vi "IR Emitter Test.vi"(5 "Test Config":T1={"Chopper RPM"=140, "IR Power"=5, "Conc Tolerance"=0.0, "Gas Stable Time"=0, "A-D Settle"=0, "Samples"=0, "Filter Time"=0, "Gas Mixtures"=[], "Filter Sequences"=[], "Functional Test"={"Mic Test ON ADC Max"=0.0, "Mic Test ON ADC Min"=0.0, "Mic Test OFF ADC Max"=0.0, "Mic Test OFF ADC Min"=0.0, "Mic Test IC ADC Max"=0.0, "Mic Test IC ADC Min"=0.0, "IR Emitter ON ADC Max"=0.0, "IR Emitter ON ADC Min"=0.0, "IR Emitter OFF ADC Max"=0.0, "IR Emitter OFF ADC Min"=0.0}, "Initial Flow Rate"=0.0, "Max Flow Rate"=0.0} {"Gas Mixtures"."ADC Gains" items=["0"=0, "3"=3, "4"=4, "5"=5, "6"=6, "7"=7]; "Conc Tolerance" min=0.0 max=100.0 step=1.0; "IR Power" min=2 max=5 step=1; "Chopper RPM" min=140 max=1000 step=1}, 8 "error in (no error)":errorcluster, 11 "Session Handle in":T6) -> (0 "error out":errorcluster, 1 "Failure Reason":string, 2 "Passed?":bool, 3 "Session Handle out":T6)   [LabVIEW 2015, in "PAS.lvclass"]
uses:
  PAS.lvclass
  Typedefs/Session Handle.ctl
  Tests/Controls/Test Config.ctl
  Tests/Controls/Gas Mixture.ctl
  Typedefs/ADC Gains.ctl
  Tests/Controls/Filter Sequence.ctl
  Tests/Controls/Functional Test.ctl
  Typedefs/Emitter Power.ctl
  Typedefs/Valves.ctl
panel:
  out "Passed?":bool
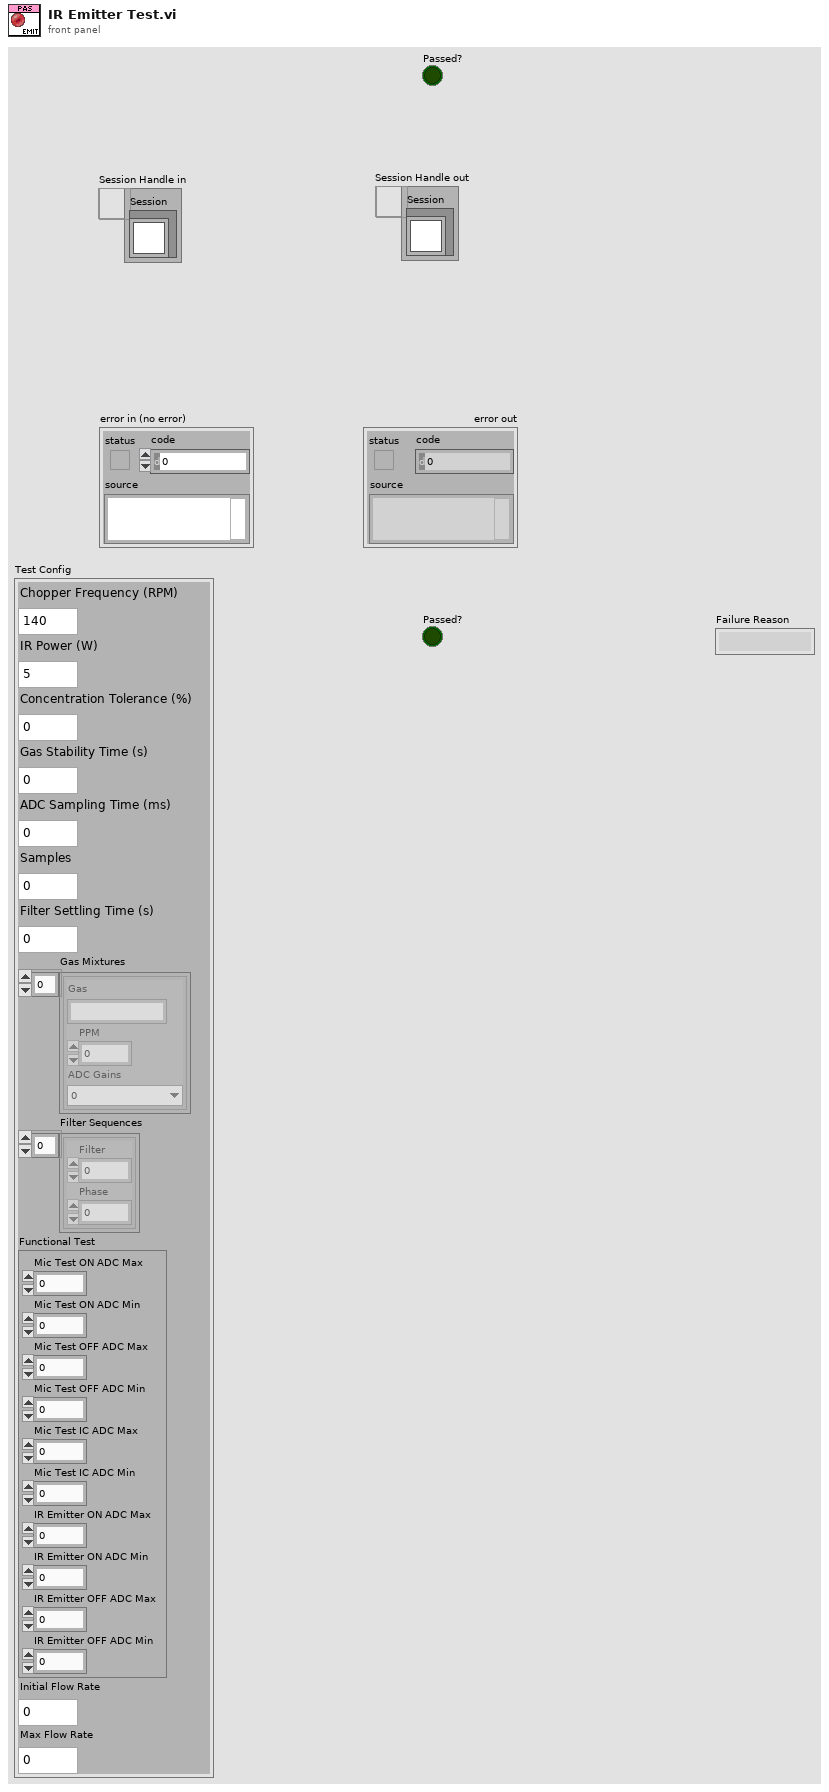
[diagram p1: front panel]
types:
  T1 = typedef "Test Config.ctl" = cluster{"Chopper RPM":u16, "IR Power":u8, "Conc Tolerance":dbl, "Gas Stable Time":u16, "A-D Settle":u16, "Samples":u16, "Filter Time":u16, "Gas Mixtures":T2[], "Filter Sequences":T4[], "Functional Test":T5, "Initial Flow Rate":sgl, "Max Flow Rate":sgl}
  T2 = typedef "Gas Mixture.ctl" = cluster{"Gas":string, "PPM":dbl, "ADC Gains":T3}
  T3 = typedef "PAS.lvclass/ADC Gains.ctl" = u16
  T4 = typedef "Filter Sequence.ctl" = cluster{"Filter":u8, "Phase":dbl}
  T5 = typedef "Functional Test.ctl" = cluster{"Mic Test ON ADC Max":dbl, "Mic Test ON ADC Min":dbl, "Mic Test OFF ADC Max":dbl, "Mic Test OFF ADC Min":dbl, "Mic Test IC ADC Max":dbl, "Mic Test IC ADC Min":dbl, "IR Emitter ON ADC Max":dbl, "IR Emitter ON ADC Min":dbl, "IR Emitter OFF ADC Max":dbl, "IR Emitter OFF ADC Min":dbl}
  T6 = typedef "PAS.lvclass/Session Handle.ctl" = refnum<data-value>
  T7 = typedef "PAS.lvclass/Valves.ctl" = u16
  T8 = typedef "PAS.lvclass/Emitter Power.ctl" = u16
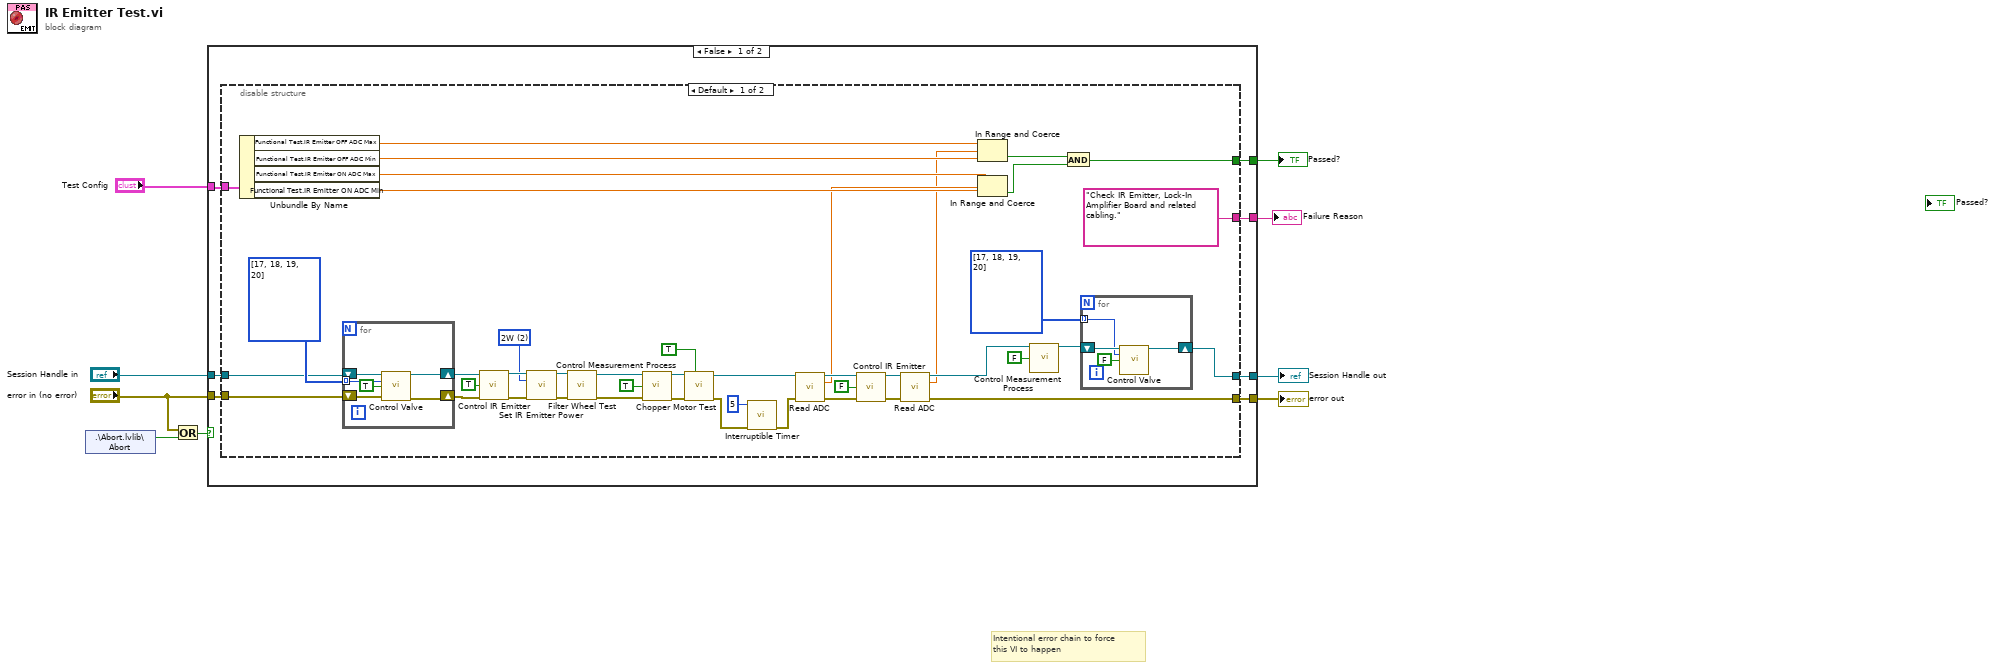
[diagram p0: block diagram]
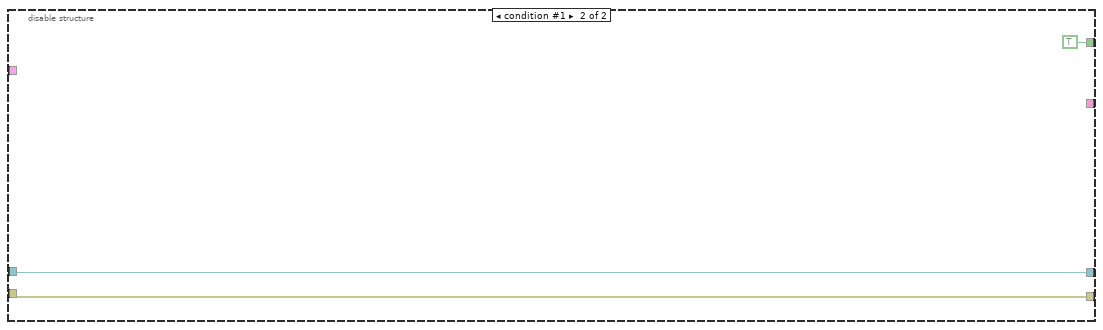
[diagram p2: hidden frame]
diagram:
  # "Intentional error chain to force\nthis VI to happen"
  n1 = shared-variable ".\\Abort.lvlib\\Abort"() -> (w4:bool)  [unwired: 1 in, 1 out]
  n2 = Or(x="error in (no error)", y=w4) -> (x .or. y?=w5:bool)
  n3 = case shown="False" w5 {
    tunnel: "error in (no error)" -> [w16 w73]
    tunnel: [w15 w74] -> w9
    tunnel: "Session Handle in" -> [w14 w74]
    tunnel: "Test Config" -> [w13 _]
    tunnel: [w12 w73] -> w7
    tunnel: [w11 _] -> w6
    tunnel: [w10 _] -> w2
    frame False {
      n4 = disable-structure shown="Default" {
        disable-tunnel: w16 -> [w59 w72]
        disable-tunnel: [w49 w71] -> w15
        disable-tunnel: w14 -> [w48 w71]
        disable-tunnel: w13 -> [w47 _]
        disable-tunnel: [w27 w72] -> w12
        disable-tunnel: [w18 TRUE] -> w11
        disable-tunnel: ["Check IR Emitter, Lock-In Amplifier Board and related cabling." ("t") _] -> w10
        frame condition #0 (active) {
          w29 = T7[] [17, 18, 19, 20] items=["PV1"=17, "PV2"=18, "PV3"=19, "PV4"=20]
          w52 = T8 2 items=["2W"=2, "3W"=3, "4W"=4, "5W"=5] ("Emitter Power")
          w58 = T7[] [17, 18, 19, 20] items=["PV1"=17, "PV2"=18, "PV3"=19, "PV4"=20]
          n5 = Unbundle By Name(w47) -> ("Functional Test.IR Emitter OFF ADC Max"=w23:dbl, "Functional Test.IR Emitter OFF ADC Min"=w22:dbl, "Functional Test.IR Emitter ON ADC Max"=w26:dbl, "Functional Test.IR Emitter ON ADC Min"=w25:dbl)
          n6 = for {
            shift-right: [w65] -> w57
            shift-left: w48 -> [w69]
            shift-right: [w66] -> w56
            shift-left: w59 -> [w67]
            tunnel: w58 -> [w68] mode=indexing
            n7 = call "Control Valve.vi"("Session Handle in"=w69, "Valves"=w68, "Energize?"=TRUE, "error in (no error)"=w67) -> ("Session Handle out"=w65:T6, "error out"=w66:errorcluster)  [unwired: 8 in, 2 out]
          }
          n8 = call "Control IR Emitter.vi"("Session Handle in"=w57, "Start?"=TRUE, "error in (no error)"=w56) -> ("Session Handle out"=w54:T6, "error out"=w53:errorcluster)  [unwired: 9 in, 2 out]
          n9 = call "Set IR Emitter Power.vi"("Session Handle in"=w54, "Emitter Power"=w52, "error in (no error)"=w53) -> ("Session Handle out"=w46:T6, "error out"=w45:errorcluster)  [unwired: 10 in, 1 out]
          n10 = call "Filter Wheel Test.vi"("error in (no error)"=w45, "Session Handle in"=w46) -> ("error out"=w36:errorcluster, "Session Handle out"=w37:T6)  [unwired: 7 in, 1 out]
          n11 = call "Control Measurement Process.vi"("Session Handle in"=w37, "Start?"=TRUE, "error in (no error)"=w36) -> ("Session Handle out"=w43:T6, "error out"=w42:errorcluster)  [unwired: 9 in, 2 out]
          n12 = call "Chopper Motor Test.vi"("Measurement Started?"=TRUE, "error in (no error)"=w42, "Session Handle in"=w43) -> ("error out"=w41:errorcluster, "Session Handle out"=w38:T6)  [unwired: 6 in, 1 out]
          n13 = call "Interruptible Timer.vi"("error in (no error)"=w41, "Wait (s)"=5) -> ("error out"=w39:errorcluster)  [unwired: 7 in, 2 out]
          n14 = call "Read ADC.vi"("Session Handle in"=w38, "error in (no error)"=w39) -> ("Session Handle out"=w34:T6, "ADC"=w24:dbl, "error out"=w33:errorcluster)  [unwired: 9 in, 2 out]
          n15 = call "Control IR Emitter.vi"("Session Handle in"=w34, "Start?"=FALSE, "error in (no error)"=w33) -> ("Session Handle out"=w31:T6, "error out"=w30:errorcluster)  [unwired: 9 in, 2 out]
          n16 = call "Read ADC.vi"("Session Handle in"=w31, "error in (no error)"=w30) -> ("Session Handle out"=w28:T6, "ADC"=w21:dbl, "error out"=w27:errorcluster)  [unwired: 9 in, 2 out]
          n17 = In Range and Coerce(upper limit=w23, x=w21, lower limit=w22) -> (In Range?=w20:bool)  [unwired: 1 out]
          n18 = In Range and Coerce(upper limit=w26, x=w24, lower limit=w25) -> (In Range?=w19:bool)  [unwired: 1 out]
          n19 = call "Control Measurement Process.vi"("Session Handle in"=w28, "Start?"=FALSE) -> ("Session Handle out"=w50:T6)  [unwired: 10 in, 3 out]
          n20 = And(x=w20, y=w19) -> (x .and. y?=w18:bool)
          n21 = for {
            shift-right: [w62] -> w49
            shift-left: w50 -> [w63]
            tunnel: w29 -> [w60] mode=indexing
            n22 = call "Control Valve.vi"("Session Handle in"=w63, "Valves"=w60, "Energize?"=FALSE) -> ("Session Handle out"=w62:T6)  [unwired: 9 in, 3 out]
          }
        }
        frame condition #1 {
        }
      }
    }
    frame True {
    }
  }
  "error out" <- w7
  "Session Handle out" <- w9
  "Passed?" <- w6
  "Failure Reason" <- w2
